vi "Aquisition_Reactor_Coolant_Loop Temperature_SG_Inlet_Average.vi"(0 "SI101_AverageReactorCoolantTemperature.lvclass":refnum<class "AverageReactorCoolantTemperature.lvclass">, 1 "3 JEC10 CT001B XQ01":dbl, 2 "3 JEC20 CT001B XQ01":dbl, 3 "3 JEC30 CT001B XQ01":dbl, 4 "3 JEC40 CT001B XQ01":dbl, 5 "error in (no error)":errorcluster) -> (14 "SI101_AverageReactorCoolantTemperature.lvclass out":refnum<class "AverageReactorCoolantTemperature.lvclass">, 15 "ACT Loop 1":dbl, 16 "ACT Loop 2":dbl, 17 "ACT loop 3":dbl, 18 "ACT loop 4":dbl, 19 "error IO":errorcluster)   [LabVIEW 2022 SP3, in "AverageReactorCoolantTemperature.lvclass"]
uses:
  AverageReactorCoolantTemperature.lvclass
  AverageReactorCoolantTemperature.lvclass/AverageReactorCoolantTemperature.ctl
panel:
  # "SI101"
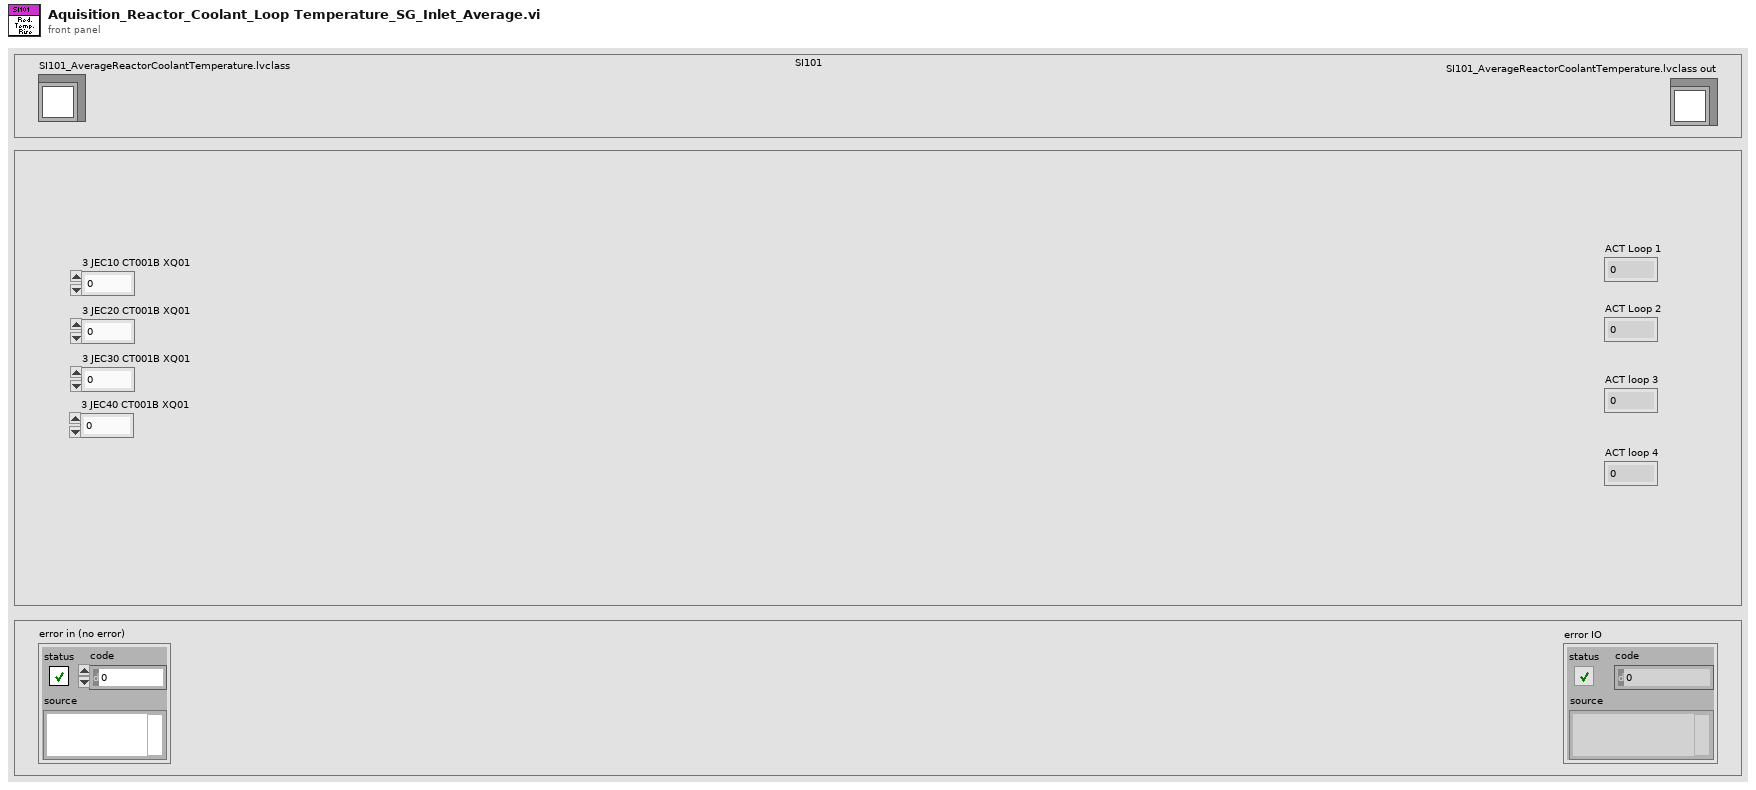
[diagram p1: front panel]
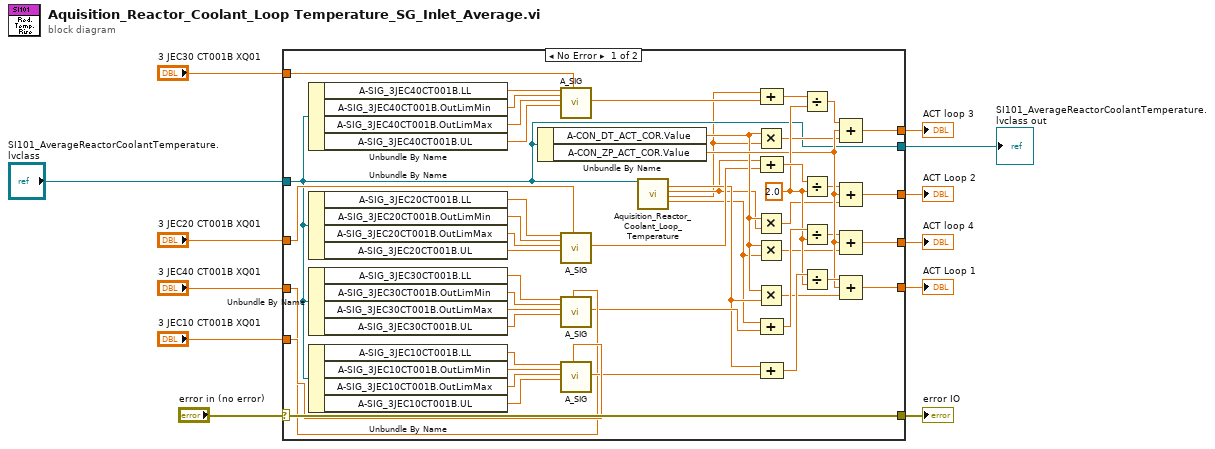
[diagram p0: block diagram]
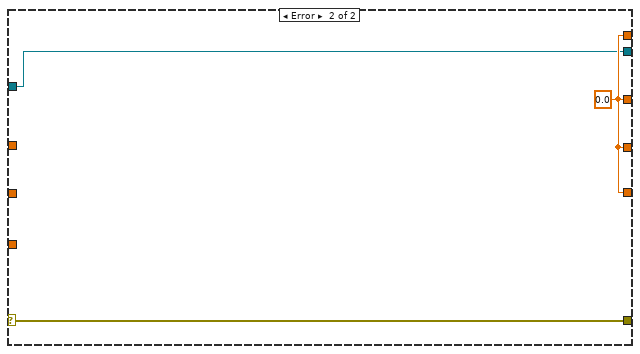
[diagram p2: hidden frame]
diagram:
  n1 = case shown="No Error" "error in (no error)" {
    selector: "error in (no error)" -> [w61 w63]
    tunnel: [w44 w64] -> w11
    tunnel: [w43 w64] -> w10
    tunnel: [w45 w64] -> w9
    tunnel: [w42 w64] -> w8
    tunnel: [w61 w63] -> w7
    tunnel: "3 JEC10 CT001B XQ01" -> [w39 _]
    tunnel: "3 JEC20 CT001B XQ01" -> [w37 _]
    tunnel: "3 JEC30 CT001B XQ01" -> [w41 _]
    tunnel: "3 JEC40 CT001B XQ01" -> [w35 _]
    tunnel: [w17 w62] -> w2
    tunnel: "SI101_AverageReactorCoolantTemperature.lvclass" -> [w17 w62]
    frame No Error {
      w56 = 2.0
      n2 = Unbundle By Name(w17) -> ("A-SIG_3JEC40CT001B.LL"=w21:dbl, "A-SIG_3JEC40CT001B.OutLimMin"=w20:dbl, "A-SIG_3JEC40CT001B.OutLimMax"=w19:dbl, "A-SIG_3JEC40CT001B.UL"=w18:dbl)
      n3 = Unbundle By Name(w17) -> ("A-SIG_3JEC20CT001B.LL"=w29:dbl, "A-SIG_3JEC20CT001B.OutLimMin"=w28:dbl, "A-SIG_3JEC20CT001B.OutLimMax"=w27:dbl, "A-SIG_3JEC20CT001B.UL"=w26:dbl)
      n4 = Unbundle By Name(w17) -> ("A-SIG_3JEC30CT001B.LL"=w25:dbl, "A-SIG_3JEC30CT001B.OutLimMin"=w24:dbl, "A-SIG_3JEC30CT001B.OutLimMax"=w23:dbl, "A-SIG_3JEC30CT001B.UL"=w22:dbl)
      n5 = Unbundle By Name(w17) -> ("A-SIG_3JEC10CT001B.LL"=w33:dbl, "A-SIG_3JEC10CT001B.OutLimMin"=w32:dbl, "A-SIG_3JEC10CT001B.OutLimMax"=w31:dbl, "A-SIG_3JEC10CT001B.UL"=w30:dbl)
      n6 = Unbundle By Name(w17) -> ("A-CON_DT_ACT_COR.Value"=w49:dbl, "A-CON_ZP_ACT_COR.Value"=w54:dbl)
      n7 = call "A_SIG.vi"("LL"=w21, "OutLimMin"=w20, "OutLimMax"=w19, "UL"=w18, "Input"=w41) -> ("A_SIG_out"=w40:dbl)  [unwired: 13 in, 1 out]
      n8 = call "A_SIG.vi"("LL"=w29, "OutLimMin"=w28, "OutLimMax"=w27, "UL"=w26, "Input"=w37) -> ("A_SIG_out"=w36:dbl)  [unwired: 13 in, 1 out]
      n9 = call "A_SIG.vi"("LL"=w25, "OutLimMin"=w24, "OutLimMax"=w23, "UL"=w22, "Input"=w35) -> ("A_SIG_out"=w34:dbl)  [unwired: 13 in, 1 out]
      n10 = call "A_SIG.vi"("LL"=w33, "OutLimMin"=w32, "OutLimMax"=w31, "UL"=w30, "Input"=w39) -> ("A_SIG_out"=w38:dbl)  [unwired: 13 in, 1 out]
      n11 = call "Aquisition_Reactor_Coolant_Loop_Temperature.vi"("SI101_AverageReactorCoolantTemperature.lvclass in"=w17) -> ("JEC10CT001A"=w16:dbl, "JEC20CT001A"=w15:dbl, "JEC30CT001A"=w14:dbl, "JEC40CT001A"=w13:dbl)  [unwired: 13 in, 2 out]
      n12 = Multiply(x=w49, y=w14) -> (x*y=w47:dbl)
      n13 = Multiply(x=w49, y=w15) -> (x*y=w48:dbl)
      n14 = Multiply(x=w49, y=w13) -> (x*y=w46:dbl)
      n15 = Multiply(x=w49, y=w16) -> (x*y=w50:dbl)
      n16 = Compound Arithmetic op=ADD(w14, w40) -> (w58:dbl)
      n17 = Compound Arithmetic op=ADD(w15, w36) -> (w59:dbl)
      n18 = Compound Arithmetic op=ADD(w13, w34) -> (w57:dbl)
      n19 = Compound Arithmetic op=ADD(w16, w38) -> (w60:dbl)
      n20 = Divide(x=w58, y=w56) -> (x/y=w52:dbl)
      n21 = Divide(x=w59, y=w56) -> (x/y=w53:dbl)
      n22 = Divide(x=w57, y=w56) -> (x/y=w51:dbl)
      n23 = Divide(x=w60, y=w56) -> (x/y=w55:dbl)
      n24 = Compound Arithmetic op=ADD(w52, w54, w47) -> (w45:dbl)
      n25 = Compound Arithmetic op=ADD(w53, w54, w48) -> (w43:dbl)
      n26 = Compound Arithmetic op=ADD(w51, w54, w46) -> (w42:dbl)
      n27 = Compound Arithmetic op=ADD(w55, w54, w50) -> (w44:dbl)
    }
    frame Error {
      w64 = 0.0 ("ACT loop n")
    }
  }
  "ACT Loop 1" <- w11
  "ACT Loop 2" <- w10
  "ACT loop 3" <- w9
  "ACT loop 4" <- w8
  "error IO" <- w7
  "SI101_AverageReactorCoolantTemperature.lvclass out" <- w2
